vi "clear queue invalid error.vi"(8 "error in":errorcluster) -> (0 "error out":errorcluster)   [LabVIEW 2023, in "Publisher Subscriber.lvlib"]
uses:
  <userlib>/_Publisher Subscriber/Publisher Subscriber.lvlib
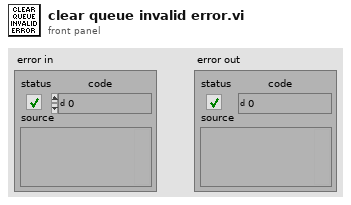
[diagram p1: front panel]
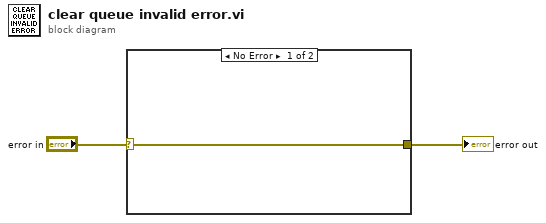
[diagram p0: block diagram]
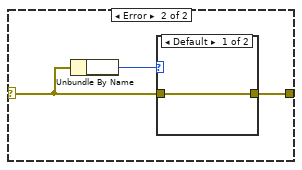
[diagram p2: hidden frame]
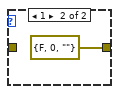
[diagram p3: hidden frame]
diagram:
  n1 = case shown="No Error" "error in" {
    selector: "error in" -> [w3 w4]
    tunnel: [w3 w5] -> w1
    frame No Error {
    }
    frame Error {
      n2 = Unbundle By Name(w4) -> (w6:i32)
      n3 = case shown="Default" w6 {
        tunnel: [w7 errorcluster {"status"=FALSE, "code"=0, "source"=""} ("error IO")] -> w5
        tunnel: w4 -> [w7 _]
        frame Default {
        }
        frame 1 {
        }
      }
    }
  }
  "error out" <- w1
